vi "getLibraryPath.vi"(8 "error in (no error)":errorcluster, 11 "ProgrammaticInitialization in":refnum<class "ProgrammaticInitialization.lvclass">) -> (0 "error out":errorcluster, 2 "SAL_Library":string, 3 "ProgrammaticInitialization out":refnum<class "ProgrammaticInitialization.lvclass">)   [LabVIEW 2016, in "ProgrammaticInitialization.lvclass"]
uses:
  ProgrammaticInitialization.lvclass
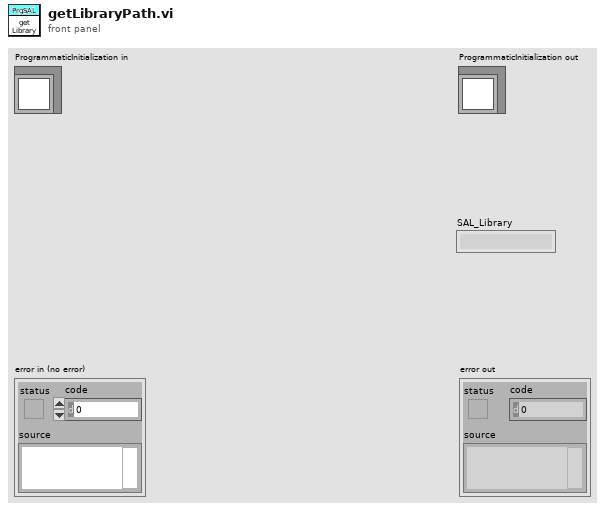
[diagram p1: front panel]
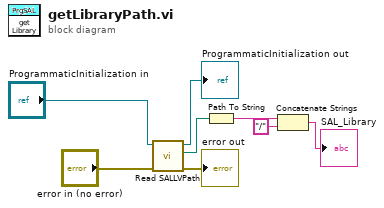
[diagram p0: block diagram]
diagram:
  n1 = call-dynamic "Read SALLVPath.vi"("error in (no error)"="error in (no error)", "ProgrammaticInitialization in"="ProgrammaticInitialization in") -> ("error out"=→"error out":errorcluster, "SALLVPath"=w4:path, "ProgrammaticInitialization out"=→"ProgrammaticInitialization out":refnum<class "ProgrammaticInitialization.lvclass">)  [unwired: 7 in]
  n2 = Path To String(path=w4) -> (string=w5:string)
  n3 = Concatenate Strings(w5, "/" ("string")) -> (→"SAL_Library":string)
